vi "Fit VI window to Rect.vi"(4 "Error In":errorcluster, 6 "Rect":T1, 7 "VI Ref":refnum<vi>) -> (0 "Error Out":errorcluster, 3 "dup VI Ref":refnum<vi>)   [LabVIEW 2017, in "csm-ui-support.lvlib"]
doc: "This VI is designed to center a callee VI's window in a caller VI's window.\n\nAuthored by Brandon Steele\nsupport@mooregoodideas.com\nwww.mooregoodideas.com\n\nCopyright (c) 2010, Moore Good Ideas, Inc.\n\nAll rights reserved.\n\nRedistribution and use in source and binary forms, with or without modification, are permitted provided that the following conditions are met:\n\n * Redistributions of source code must retain the above copyright notice, this list of conditions and the following disclaimer.\n * Redistributions in binary form must reproduce the above copyright notice, this list of conditions and the following disclaimer in the documentation and/or other materials provided with the distribution.\n * Neither the name of Moore Good Ideas, Inc. nor the names of its contributors may be used to endorse or promote products derived from this software without specific prior written permission.\n\nTHIS SOFTWARE IS PROVIDED BY THE COPYRIGHT HOLDERS AND CONTRIBUTORS \"AS IS\" AND ANY EXPRESS OR IMPLIED WARRANTIES, INCLUDING, BUT NOT LIMITED TO, THE IMPLIED WARRANTIES OF MERCHANTABILITY AND FITNESS FOR A PARTICULAR PURPOSE ARE DISCLAIMED. IN NO EVENT SHALL THE COPYRIGHT OWNER OR CONTRIBUTORS BE LIABLE FOR ANY DIRECT, INDIRECT, INCIDENTAL, SPECIAL, EXEMPLARY, OR CONSEQUENTIAL DAMAGES (INCLUDING, BUT NOT LIMITED TO, PROCUREMENT OF SUBSTITUTE GOODS OR SERVICES; LOSS OF USE, DATA, OR PROFITS; OR BUSINESS INTERRUPTION) HOWEVER CAUSED AND ON ANY THEORY OF LIABILITY, WHETHER IN CONTRACT, STRICT LIABILITY, OR TORT (INCLUDING NEGLIGENCE OR OTHERWISE) ARISING IN ANY WAY OUT OF THE USE OF THIS SOFTWARE, EVEN IF ADVISED OF THE POSSIBILITY OF SUCH DAMAGE."
uses:
  <vilib>/Utility/miscctls.llb/LVRectTypeDef.ctl
  csm-ui-support.lvlib
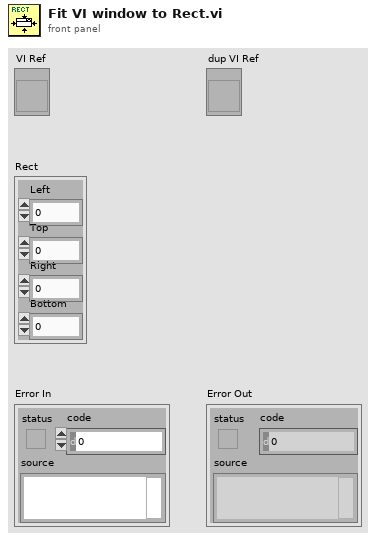
[diagram p1: front panel]
types:
  T1 = typedef "LVRectTypeDef.ctl" = cluster{"Left":i16, "Top":i16, "Right":i16, "Bottom":i16}
  T2 = cluster{"left":i16, "top":i16, "right":i16, "bottom":i16}
  T3 = typedef "LVAllMonitorsDisplayTypeDef.ctl" = cluster{"Bounds":cluster{"Left":i16, "Top":i16, "Right":i16, "Bottom":i16}, "Depth":i16}[]
  T4 = cluster{"Left":i16, "Top":i16, "Right":i16, "Bottom":i16}
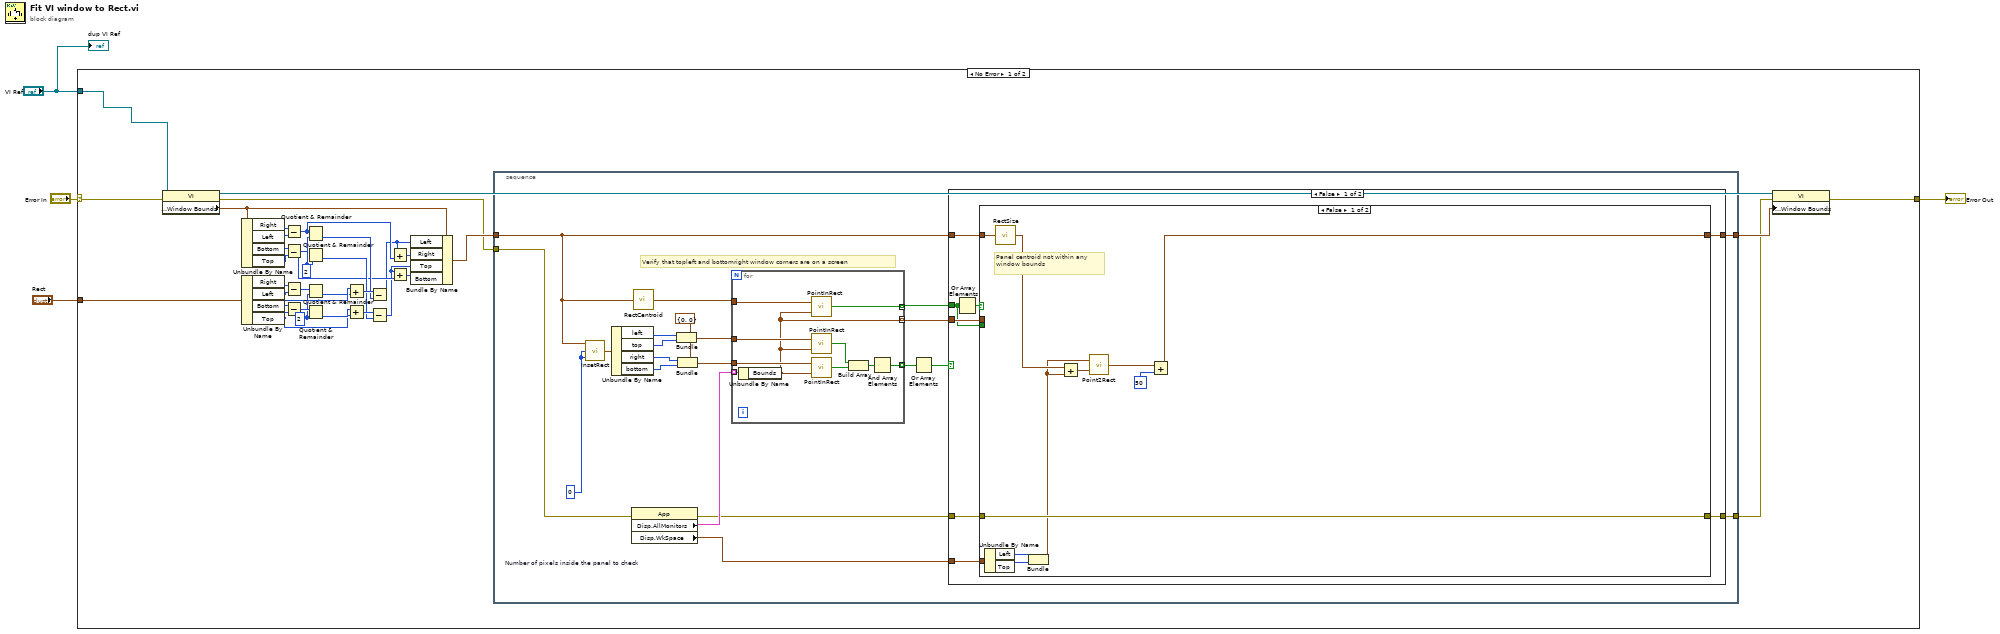
[diagram p0: block diagram]
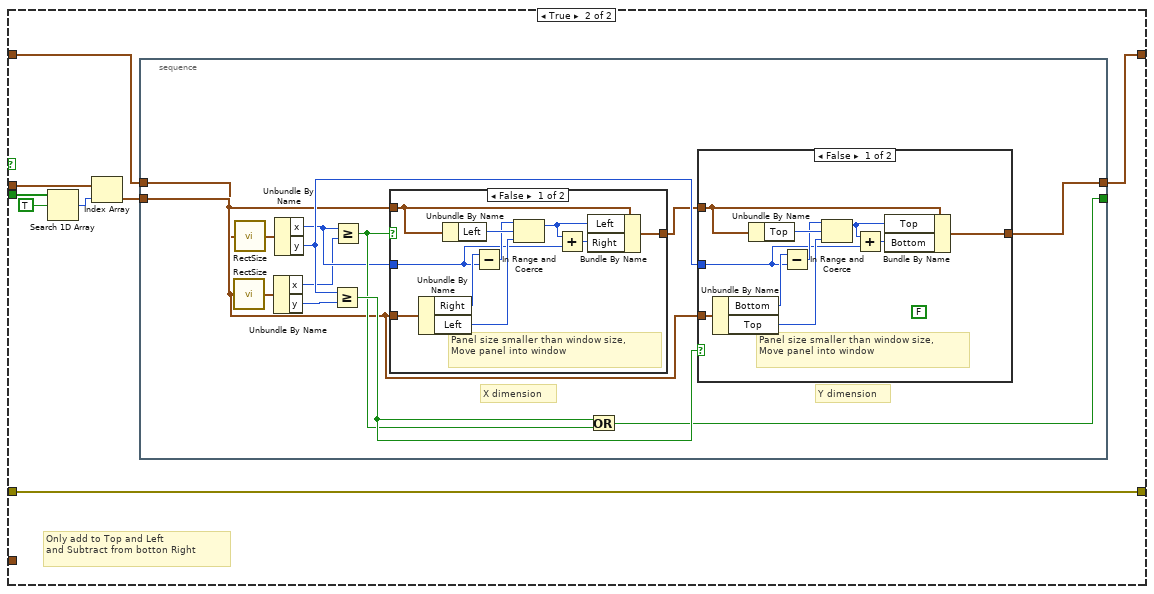
[diagram p2: hidden frame]
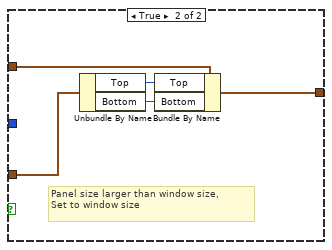
[diagram p3: hidden frame]
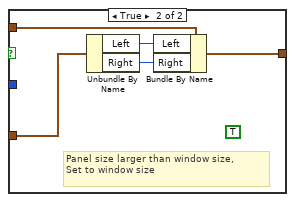
[diagram p4: hidden frame]
diagram:
  n1 = case shown="No Error" "Error In" {
    selector: "Error In" -> [w7 w142]
    tunnel: [w38 w142] -> w4
    tunnel: "VI Ref" -> [w5 _]
    tunnel: "Rect" -> [w6 _]
    frame No Error {
      w33 = i16 2 ("y")
      w17 = i16 2 ("y")
      n2 = property class="VI"(reference=w5, error in=w7) -> (reference out=w20:refnum<vi>, error out=w9:errorcluster, "Front Panel Window:Window Bounds"=w12:T1)
      n3 = Unbundle By Name(w12) -> ("Right"=w29:i16, "Left"=w30:i16, "Bottom"=w31:i16, "Top"=w32:i16)
      n4 = Unbundle By Name(w6) -> ("Right"=w37:i16, "Left"=w28:i16, "Bottom"=w36:i16, "Top"=w25:i16)
      n5 = Subtract(x=w29, y=w30) -> (x-y=w19:i16)
      n6 = Subtract(x=w31, y=w32) -> (x-y=w18:i16)
      n7 = Subtract(x=w37, y=w28) -> (x-y=w35:i16)
      n8 = Subtract(x=w36, y=w25) -> (x-y=w34:i16)
      n9 = Quotient & Remainder(x=w19, y=w33) -> (floor(x/y)=w23:i16)  [unwired: 1 out]
      n10 = Quotient & Remainder(x=w18, y=w33) -> (floor(x/y)=w21:i16)  [unwired: 1 out]
      n11 = Quotient & Remainder(x=w35, y=w17) -> (floor(x/y)=w27:i16)  [unwired: 1 out]
      n12 = Quotient & Remainder(x=w34, y=w17) -> (floor(x/y)=w26:i16)  [unwired: 1 out]
      n13 = Add(x=w28, y=w27) -> (x+y=w24:i16)
      n14 = Add(x=w25, y=w26) -> (x+y=w22:i16)
      n15 = Subtract(x=w24, y=w23) -> (x-y=w15:i16)
      n16 = Subtract(x=w22, y=w21) -> (x-y=w14:i16)
      n17 = Add(x=w15, y=w19) -> (x+y=w13:i16)
      n18 = Add(x=w14, y=w18) -> (x+y=w16:i16)
      n19 = Bundle By Name(cluster=w12, "Left"=w15, "Right"=w13, "Top"=w14, "Bottom"=w16) -> (w11:T1)
      n20 = stacked-sequence {
        tunnel: [w49] -> w8
        tunnel: [w40] -> w10
        tunnel: w9 -> [w42]
        tunnel: w11 -> [w56]
        frame #0 {
          w51 = i16 0  # Number of pixels inside the panel to check
          w55 = cluster{"x":i16, "y":i16} {"x"=0, "y"=0} ("point")
          # "Verify that topleft and bottomright window corners are on a screen"
          n21 = call <vilib>:"InsetRect.vi"("dv"=w51, "dh"=w51, "rect"=w56) -> ("inset rect"=w45:T2)
          n22 = Unbundle By Name(w45) -> ("left"=w43:i16, "top"=w44:i16, "right"=w52:i16, "bottom"=w53:i16)
          n23 = property class="App"(error in=w42) -> (error out=w39:errorcluster, "Disp.AllMonitors"=w41:T3, "Disp.WkSpace"=w50:T1)  [unwired: 1 in, 1 out]
          n24 = call <vilib>:"RectCentroid.vi"("rect"=w56) -> ("point"=w57:cluster{"x":i16, "y":i16})
          n25 = Bundle(cluster=w55, "x"=w43, "y"=w44) -> (w46:cluster{"x":i16, "y":i16})
          n26 = Bundle(cluster=w55, "x"=w52, "y"=w53) -> (w54:cluster{"x":i16, "y":i16})
          n27 = for {
            tunnel: w41 -> [w141] mode=indexing
            tunnel: w46 -> [w140]
            tunnel: [w136] -> w47 mode=indexing
            tunnel: w54 -> [w135]
            tunnel: w57 -> [w134]
            tunnel: [w133] -> w58 mode=indexing
            tunnel: [w132] -> w59 mode=indexing
            n28 = Unbundle By Name(w141) -> ("Bounds"=w132:T4)
            n29 = call <vilib>:"PointInRect.vi"("rect"=w132, "point"=w134) -> ("pt in rect"=w133:bool)
            n30 = call <vilib>:"PointInRect.vi"("rect"=w132, "point"=w140) -> ("pt in rect"=w139:bool)
            n31 = call <vilib>:"PointInRect.vi"("rect"=w132, "point"=w135) -> ("pt in rect"=w138:bool)
            n32 = Build Array(w139, w138) -> (w137:bool[])
            n33 = And Array Elements(Boolean array=w137) -> (logical AND=w136:bool)
          }
          n34 = Or Array Elements(Boolean array=w47) -> (logical OR=w48:bool)
          n35 = case shown="False" w48 {
            tunnel: w39 -> [w62 w131]
            tunnel: [w61 w131] -> w49
            tunnel: w56 -> [w66 w130]
            tunnel: [w65 w130] -> w40
            tunnel: w50 -> [w67 _]
            tunnel: w58 -> [w60 _]
            tunnel: w59 -> [w63 _]
            frame False {
              n36 = Or Array Elements(Boolean array=w60) -> (logical OR=w64:bool)
              n37 = case shown="False" w64 {
                tunnel: w67 -> [w78 _]
                tunnel: w66 -> [w74 w81]
                tunnel: [w72 w79] -> w65
                tunnel: w63 -> [_ w83]
                tunnel: w62 -> [w71 w86]
                tunnel: [w71 w86] -> w61
                tunnel: w60 -> [_ w85]
                frame False {
                  # "Panel centroid not within any\nwindow bounds"
                  n38 = Unbundle By Name(w78) -> ("Left"=w77:i16, "Top"=w76:i16)
                  n39 = call <vilib>:"RectSize.vi"("rect"=w74) -> ("point"=w70:cluster{"x":i16, "y":i16})
                  n40 = Bundle("Left"=w77, "Top"=w76) -> (w68:cluster{"Left":i16, "Top":i16})  [unwired: 1 in]
                  n41 = Add(x=w70, y=w68) -> (x+y=w69:cluster{i16, i16})
                  n42 = call <vilib>:"Point2Rect.vi"("point b"=w69, "point a"=w68) -> ("rect"=w73:T2)
                  n43 = Add(x=w73, y=i16 50) -> (x+y=w72:T2)
                }
                frame True {
                  # "Only add to Top and Left\nand Subtract from botton Right"
                  n44 = Search 1D Array(1D array=w85, element=TRUE) -> (index of element=w82:i32)  [unwired: 1 in]
                  n45 = Index Array(array=w83, index=w82) -> (element=w80:T4)
                  n46 = stacked-sequence {
                    tunnel: [w87] -> _
                    tunnel: [w97] -> w79
                    tunnel: w80 -> [w96]
                    tunnel: w81 -> [w88]
                    frame #0 {
                      # "X dimension"
                      # "Y dimension"
                      n47 = call <vilib>:"RectSize.vi"("rect"=w96) -> ("point"=w90:cluster{"x":i16, "y":i16})
                      n48 = call <vilib>:"RectSize.vi"("rect"=w88) -> ("point"=w89:cluster{"x":i16, "y":i16})
                      n49 = Unbundle By Name(w90) -> ("x"=w91:i16, "y"=w94:i16)
                      n50 = Unbundle By Name(w89) -> ("x"=w92:i16, "y"=w95:i16)
                      n51 = Greater Or Equal?(x=w95, y=w94) -> (x >= y?=w99:bool)
                      n52 = Greater Or Equal?(x=w92, y=w91) -> (x >= y?=w98:bool)
                      n53 = case shown="False" w98 {
                        tunnel: w96 -> [w124 w125]
                        tunnel: w88 -> [w116 w126]
                        tunnel: w92 -> [w117 _]
                        tunnel: [w115 w127] -> w93
                        frame False {
                          # "Panel size smaller than window size,\nMove panel into window"
                          n54 = Unbundle By Name(w124) -> ("Right"=w120:i16, "Left"=w122:i16)
                          n55 = Unbundle By Name(w116) -> ("Left"=w123:i16)
                          n56 = Subtract(x=w120, y=w117) -> (x-y=w121:i16)
                          n57 = In Range and Coerce(upper limit=w121, x=w123, lower limit=w122) -> (coerced(x)=w119:i16)  [unwired: 1 out]
                          n58 = Add(x=w119, y=w117) -> (x+y=w118:i16)
                          n59 = Bundle By Name(cluster=w116, "Left"=w119, "Right"=w118) -> (w115:T1)
                        }
                        frame True {
                          (unwired) TRUE
                          # "Panel size larger than window size,\nSet to window size"
                          n60 = Unbundle By Name(w125) -> ("Left"=w129:i16, "Right"=w128:i16)
                          n61 = Bundle By Name(cluster=w126, "Left"=w129, "Right"=w128) -> (w127:T1)
                        }
                      }
                      n62 = Or(x=w99, y=w98) -> (x .or. y?=w87:bool)
                      n63 = case shown="False" w99 {
                        tunnel: w96 -> [w109 w114]
                        tunnel: w93 -> [w101 w110]
                        tunnel: w95 -> [w102 _]
                        tunnel: [w100 w111] -> w97
                        frame False {
                          (unwired) FALSE
                          # "Panel size smaller than window size,\nMove panel into window"
                          n64 = Unbundle By Name(w109) -> ("Bottom"=w105:i16, "Top"=w107:i16)
                          n65 = Unbundle By Name(w101) -> ("Top"=w108:i16)
                          n66 = Subtract(x=w105, y=w102) -> (x-y=w106:i16)
                          n67 = In Range and Coerce(upper limit=w106, x=w108, lower limit=w107) -> (coerced(x)=w104:i16)  [unwired: 1 out]
                          n68 = Add(x=w104, y=w102) -> (x+y=w103:i16)
                          n69 = Bundle By Name(cluster=w101, "Top"=w104, "Bottom"=w103) -> (w100:T1)
                        }
                        frame True {
                          # "Panel size larger than window size,\nSet to window size"
                          n70 = Unbundle By Name(w114) -> ("Top"=w113:i16, "Bottom"=w112:i16)
                          n71 = Bundle By Name(cluster=w110, "Top"=w113, "Bottom"=w112) -> (w111:T1)
                        }
                      }
                    }
                  }
                }
              }
            }
            frame True {
            }
          }
        }
      }
      n72 = property class="VI"(reference=w20, error in=w8, "Front Panel Window:Window Bounds"=w10) -> (error out=w38:errorcluster)  [unwired: 1 out]
    }
    frame Error {
    }
  }
  "Error Out" <- w4
  "dup VI Ref" <- "VI Ref"
